vi "ReferenceFeedbackTurnedOn.vi"(8 "error in":errorcluster) -> (0 "error out":errorcluster, 2 "Mode":refnum<vi>, 3 "FeedbackOn?":refnum<vi>)   [LabVIEW 2016]
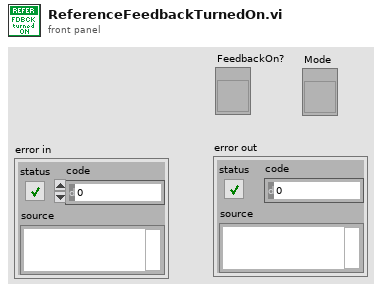
[diagram p1: front panel]
types:
  T1 = enum32{"Bad", "Idle", "Run top level", "Running"}
  T2 = enum32{"Invalid", "Standard", "Closed", "Hidden", "Minimized", "Maximized"}
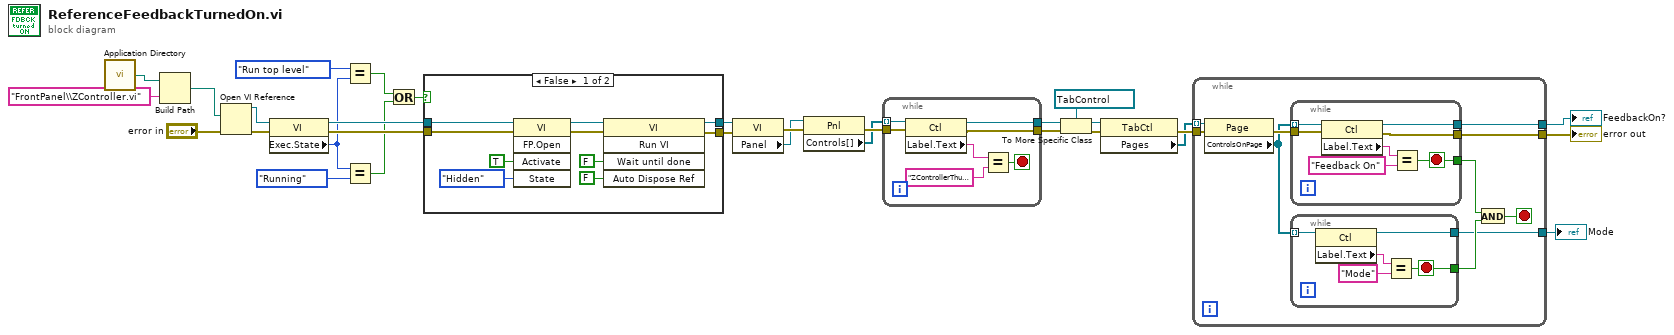
[diagram p0: block diagram]
diagram:
  n1 = call <vilib>:"Application Directory.vi"() -> ("Application Directory"=w24:path)
  n2 = Build Path(base path=w24, name or relative path="FrontPanel\\ZController.vi") -> (appended path=w23:path)
  n3 = Open VI Reference(vi path=w23, error in (no error)="error in") -> (vi reference=w2:refnum<vi>, error out=w3:errorcluster)  [unwired: 4 in]
  n4 = property class="VI"(reference=w2, error in=w3) -> (reference out=w14:refnum<vi>, error out=w13:errorcluster, "Exec.State"=w8:T1)
  n5 = Equal?(x=T1."Run top level" ("Execution:State"), y=w8) -> (x = y?=w10:bool)
  n6 = Equal?(x=w8, y=T1."Running" ("Execution:State")) -> (x = y?=w9:bool)
  n7 = Or(x=w10, y=w9) -> (x .or. y?=w7:bool)
  n8 = case shown="False" w7 {
    tunnel: [w35 w41] -> w5
    tunnel: [w34 w42] -> w4
    tunnel: w14 -> [w32 w42]
    tunnel: w13 -> [w31 w41]
    frame False {
      n9 = invoke class="VI" method="FP.Open"(reference=w32, error in=w31, "Activate"=TRUE ("Activate?"), "State"=T2."Hidden") -> (reference out=w37:refnum<vi>, error out=w36:errorcluster)  [unwired: 1 in, 3 out]
      n10 = invoke class="VI" method="Run VI"(reference=w37, error in=w36, "Wait until done"=FALSE ("Wait Until Done"), "Auto Dispose Ref"=FALSE ("Auto Dispose Reference")) -> (reference out=w34:refnum<vi>, error out=w35:errorcluster)  [unwired: 1 in, 3 out]
    }
    frame True {
    }
  }
  n11 = property class="VI"(reference=w4, error in=w5) -> (error out=w29:errorcluster, "Panel"=w22:refnum<vi>)  [unwired: 1 out]
  n12 = property class="Pnl"(reference=w22, error in=w29) -> (error out=w30:errorcluster, "Controls[]"=w26:refnum<vi>[])  [unwired: 1 out]
  n13 = while {
    tunnel: w26 -> [w49] mode=indexing
    tunnel: [w47] -> w27
    tunnel: [w46] -> w28
    tunnel: w30 -> [w45]
    stop <- w44 stop-if-true
    n14 = property class="Ctl"(reference=w49, error in=w45) -> (reference out=w47:refnum<vi>, error out=w46:errorcluster, "Label.Text"=w43:string)
    n15 = Equal?(x=w43, y="ZControllerThumbnail") -> (x = y?=w44:bool)
  }
  n16 = To More Specific Class(target class=refnum<vi> refnum ("Menus"), reference=w27, error in=w28) -> (specific class reference=w17:refnum<vi>, error out=w20:errorcluster)
  n17 = property class="TabCtl"(reference=w17, error in=w20) -> (error out=w19:errorcluster, "Pages"=w18:refnum<vi>[])  [unwired: 1 out]
  n18 = while {
    tunnel: w18 -> [w59] mode=indexing
    tunnel: [w58] -> w15
    tunnel: [w57] -> w6
    tunnel: w19 -> [w55]
    tunnel: [w50] -> w1
    stop <- w52 stop-if-true
    n19 = property class="Page"(reference=w59, error in=w55) -> (error out=w56:errorcluster, "ControlsOnPage"=w51:refnum<vi>[])  [unwired: 1 out]
    n20 = while {
      tunnel: w51 -> [w71] mode=indexing
      tunnel: [w65] -> w54
      tunnel: [w69] -> w58
      tunnel: [w68] -> w57
      tunnel: w56 -> [w67]
      stop <- w65 stop-if-true
      n21 = property class="Ctl"(reference=w71, error in=w67) -> (reference out=w69:refnum<vi>, error out=w68:errorcluster, "Label.Text"=w66:string)
      n22 = Equal?(x=w66, y="Feedback On") -> (x = y?=w65:bool)
    }
    n23 = while {
      tunnel: [w62] -> w53
      tunnel: w51 -> [w61] mode=indexing
      tunnel: [w60] -> w50
      stop <- w62 stop-if-true
      n24 = property class="Ctl"(reference=w61) -> (reference out=w60:refnum<vi>, "Label.Text"=w64:string)  [unwired: 1 in, 1 out]
      n25 = Equal?(x=w64, y="Mode") -> (x = y?=w62:bool)
    }
    n26 = And(x=w54, y=w53) -> (x .and. y?=w52:bool)
  }
  "error out" <- w6
  "FeedbackOn?" <- w15
  "Mode" <- w1
